vi "Vision_Test.vi"() -> ()   [LabVIEW 2011]
uses:
  <vilib>/Rock Robotics/WPI/Camera/WPI_CameraImageSize.ctl
  <vilib>/Platform/TimedLoop/XDataNode/timing_clust.ctl
  <vilib>/Platform/TimedLoop/XDataNode/nitl_modes.ctl
  <vilib>/Platform/TimedLoop/XDataNode/wakeup.ctl
  <vilib>/Platform/TimedLoop/XDataNode/XDataNode.xnode
  <vilib>/vision/NI_Vision_Development_Module.lvlib
  <vilib>/Platform/TimedLoop/XDataNode/XDNodeRunTimeDep.lvlib
panel:
  out "Wait":bool
  in  "Image Res":T1=enum."320x240"
  out "Offset_Angle_From_Perpendicular":dbl
  out "Shortest_Dist_To_Rect_Center":dbl
  in  "Rect_Width":dbl=24.0
  out "Processed Image":T2(plugin-control)
  out "Raw 2":T2(plugin-control)
  out "Raw 1":T2(plugin-control)
  in  "Threshold Range":cluster{"Lower value":sgl, "Upper value":sgl}={"Lower value"=240.0, "Upper value"=255.0} {"Upper value" format="%.2f"; "Lower value" format="%.2f"}
  out "Image 2":T2(plugin-control)
  out "Image 1":T2(plugin-control)
  in  "Milsec Wait":u32=3000
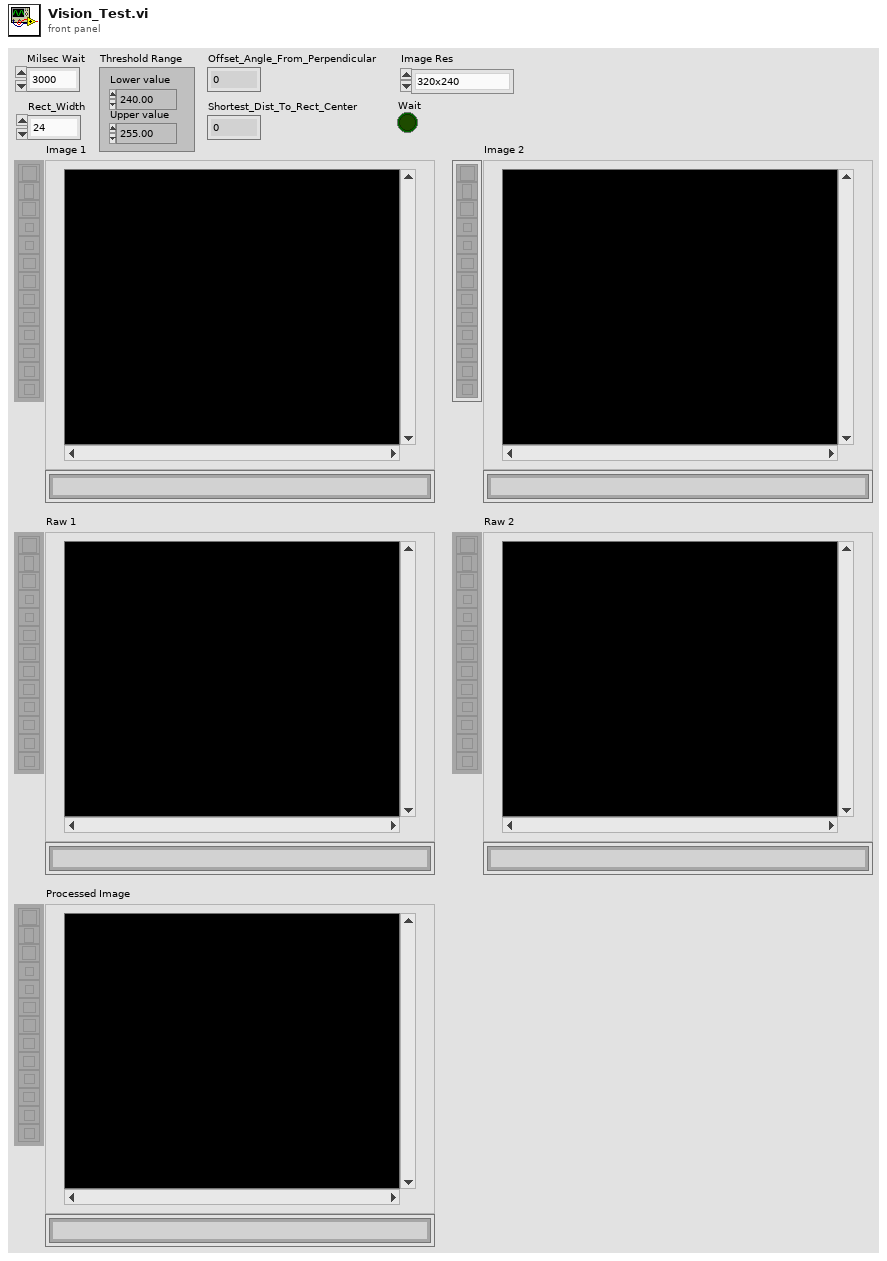
[diagram p1: front panel]
types:
  T1 = typedef "WPI_CameraImageSize.ctl" = enum16{"640x480", "320x240", "160x120"}
  T2 = typedef "IMAQ Image.ctl" = refnum<image>
  T3 = typedef "Image Type" = u32
  T4 = typedef "WPI_CameraDevRef.ctl" = cluster{"Camera Address":string, "CameraStatus":errorcluster, "Acquire Image Notifier":refnum<notifier>}
  T5 = typedef "XDNodeRunTimeDep.lvlib/timing_clust.ctl" = cluster{"Expected End [f-1]":u64, "Actual End [f-1]":u64, "Finished Late? [f-1]":bool, "Expected End [i-1]":u64, "Actual End [i-1]":u64, "Finished Late? [i-1]":bool, "Expected Start [i]":u64, "Actual Start [i]":u64, "Expected Start [f]":u64, "Actual Start [f]":u64, "Source Name":string, "Structure Name":string, "Period":i64, "Deadline":i64, "Offset":i64, "Start":i64, "Priority":i32, "Timeout":i32, "Mode":T6, "Wakeup Reason":T7, "Error":errorcluster, "Source Type":string, "Secondary Source Type":string, "Global End Time":u64, "Global Start Time":u64, "Frame Duration":u64, "Iteration Duration":u64, "Assigned CPU":i32, "I/O Scan Engine Mode":u32}
  T6 = typedef "XDNodeRunTimeDep.lvlib/nitl_modes.ctl" = enum32{"No Change", "Process missed periods, maintain original phase", "Discard missed periods, maintain original phase", "Process missed periods, ignore original phase", "Discard missed periods, ignore original phase"}
  T7 = typedef "XDNodeRunTimeDep.lvlib/wakeup.ctl" = enum32{"Normal", "Aborted", "Asynchronous wakeup", "Timing source error", "Timed loop error", "Timeout"}
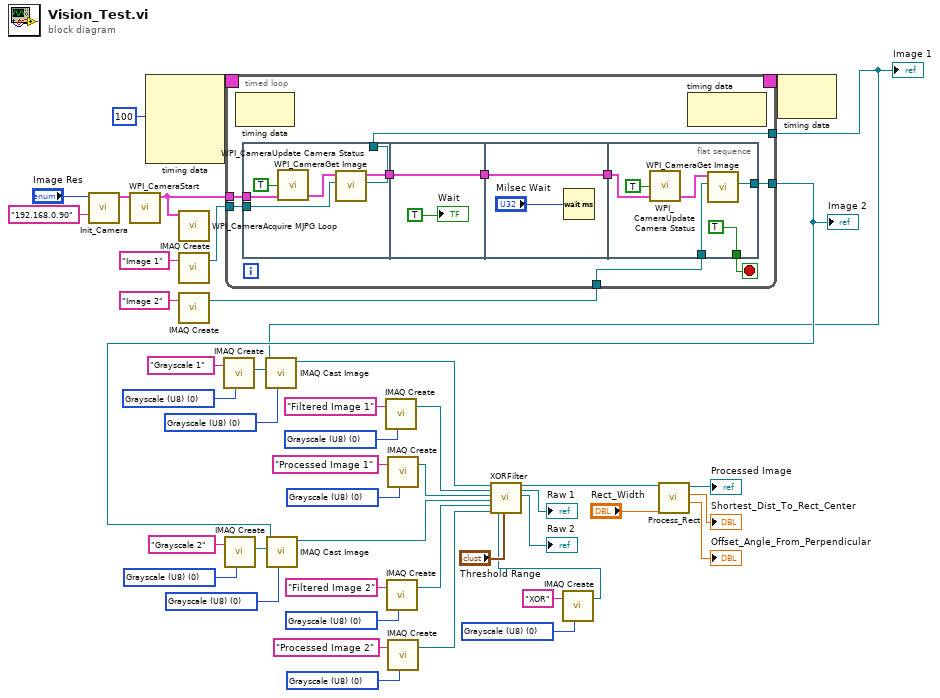
[diagram p0: block diagram]
diagram:
  w17 = T3 0 items=["Grayscale (U8)", "Grayscale (I16)", "Grayscale (SGL)", "Complex (CSG)", "RGB (U32)", "HSL (U32)", "RGB (U64)", "Grayscale (U16)"] ("Image Type")
  w28 = T3 0 items=["Grayscale (U8)", "Grayscale (I16)", "Grayscale (SGL)", "Complex (CSG)", "RGB (U32)", "HSL (U32)", "RGB (U64)", "Grayscale (U16)"] ("Image Type")
  w27 = T3 0 items=["Grayscale (U8)", "Grayscale (I16)", "Grayscale (SGL)", "Complex (CSG)", "RGB (U32)", "HSL (U32)", "RGB (U64)", "Grayscale (U16)"] ("Image Type")
  w29 = T3 0 items=["Grayscale (U8)", "Grayscale (I16)", "Grayscale (SGL)", "Complex (CSG)", "RGB (U32)", "HSL (U32)", "RGB (U64)", "Grayscale (U16)"] ("Image Type")
  w30 = T3 0 items=["Grayscale (U8)", "Grayscale (I16)", "Grayscale (SGL)", "Complex (CSG)", "RGB (U32)", "HSL (U32)", "RGB (U64)", "Grayscale (U16)"] ("Image Type")
  w34 = T3 0 items=["Grayscale (U8)", "Grayscale (I16)", "Grayscale (SGL)", "Complex (CSG)", "RGB (U32)", "HSL (U32)", "RGB (U64)", "Grayscale (U16)"] ("Image Type")
  w35 = T3 0 items=["Grayscale (U8)", "Grayscale (I16)", "Grayscale (SGL)", "Complex (CSG)", "RGB (U32)", "HSL (U32)", "RGB (U64)", "Grayscale (U16)"] ("Image Type")
  w38 = T3 0 items=["Grayscale (U8)", "Grayscale (I16)", "Grayscale (SGL)", "Complex (CSG)", "RGB (U32)", "HSL (U32)", "RGB (U64)", "Grayscale (U16)"] ("Image Type")
  w39 = T3 0 items=["Grayscale (U8)", "Grayscale (I16)", "Grayscale (SGL)", "Complex (CSG)", "RGB (U32)", "HSL (U32)", "RGB (U64)", "Grayscale (U16)"] ("Image Type")
  n1 = call "Init_Camera.vi"("Camera IP"="192.168.0.90", "Image Size"="Image Res") -> ("CameraDevRef Out"=w46:T4)  [unwired: 9 in]
  n2 = call <vilib>:"WPI_CameraStart.vi"("CameraDevRef"=w46) -> ("CameraDevRef Out"=w45:T4)  [unwired: 9 in, 1 out]
  n3 = node-c288(i64 100 ("Period")) -> (w8:T5)  [unwired: 3 in]
  n4 = call <vilib>:"WPI_CameraAcquire MJPG Loop.vi"("CameraDevRef"=w45) -> ()  [unwired: 11 in]
  n5 = call "IMAQ Create"("Image Name"="Image 1") -> ("New Image"=w42:T2)  [unwired: 4 in, 1 out]
  n6 = call "IMAQ Create"("Image Name"="Image 2") -> ("New Image"=w41:T2)  [unwired: 4 in, 1 out]
  n7 = call "IMAQ Create"("Image Name"="Grayscale 1", "Image Type"=w30) -> ("New Image"=w32:T2)  [unwired: 3 in, 1 out]
  n8 = call "IMAQ Create"("Image Name"="Grayscale 2", "Image Type"=w27) -> ("New Image"=w25:T2)  [unwired: 3 in, 1 out]
  n9 = timed-loop {
    tunnel: w45 -> [w54]
    tunnel: w42 -> [w53]
    tunnel: w41 -> [w52]
    tunnel: [w50] -> w24
    timing: w8 -> [_]
    timing-out: [_] -> w7
    tunnel: [w47] -> w4
    stop <- w51 stop-if-true
    n10 = node-c288() -> ()  [unwired: 1 in, 1 out]
    n11 = flat-sequence {
      tunnel: [w61] -> w49
      tunnel: w54 -> [w60]
      tunnel: w53 -> [w59]
      tunnel: [w58] -> _
      tunnel: [w58] -> w47
      tunnel: w49 -> [w65]
      tunnel: [w65] -> w48
      tunnel: [w66] -> w55
      tunnel: w48 -> [w66]
      tunnel: w55 -> [w71]
      tunnel: w52 -> [w70]
      tunnel: [TRUE] -> w51
      tunnel: [w68] -> w50
      frame #0 {
        n12 = call <vilib>:"WPI_CameraUpdate Camera Status.vi"("CameraDevRef In"=w60, "Enable Vision"=TRUE) -> ("CameraDevRef Out"=w63:T4)  [unwired: 3 in]
        n13 = call <vilib>:"WPI_CameraGet Image.vi"("Image"=w59, "CameraDevRef"=w63) -> ("Image Out"=w58:T2, "CameraDevRef Out"=w61:T4)  [unwired: 7 in, 1 out]
      }
      frame #1 {
        "Wait" <- TRUE
      }
      frame #2 {
        n14 = Wait (ms)(milliseconds to wait="Milsec Wait") -> ()  [unwired: 1 out]
      }
      frame #3 {
        n15 = call <vilib>:"WPI_CameraUpdate Camera Status.vi"("CameraDevRef In"=w71, "Enable Vision"=TRUE) -> ("CameraDevRef Out"=w72:T4)  [unwired: 3 in]
        n16 = call <vilib>:"WPI_CameraGet Image.vi"("Image"=w70, "CameraDevRef"=w72) -> ("Image Out"=w68:T2)  [unwired: 7 in, 2 out]
      }
    }
    n17 = node-c288() -> ()  [unwired: 1 in, 1 out]
  }
  "Image 1" <- w4
  "Image 2" <- w24
  n18 = call "IMAQ Cast Image"("Image Type"=w29, "Image Dst"=w32, "Image Src"=w4) -> ("Image Dst Out"=w23:T2)  [unwired: 7 in, 1 out]
  n19 = call "IMAQ Cast Image"("Image Type"=w28, "Image Dst"=w25, "Image Src"=w24) -> ("Image Dst Out"=w20:T2)  [unwired: 7 in, 1 out]
  n20 = call "IMAQ Create"("Image Name"="Filtered Image 1", "Image Type"=w35) -> ("New Image"=w22:T2)  [unwired: 3 in, 1 out]
  n21 = call "IMAQ Create"("Image Name"="Filtered Image 2", "Image Type"=w34) -> ("New Image"=w19:T2)  [unwired: 3 in, 1 out]
  n22 = call "IMAQ Create"("Image Name"="Processed Image 1", "Image Type"=w39) -> ("New Image"=w21:T2)  [unwired: 3 in, 1 out]
  n23 = call "IMAQ Create"("Image Name"="Processed Image 2", "Image Type"=w38) -> ("New Image"=w18:T2)  [unwired: 3 in, 1 out]
  n24 = call "IMAQ Create"("Image Name"="XOR", "Image Type"=w17) -> ("New Image"=w1:T2)  [unwired: 3 in, 1 out]
  n25 = call "XORFilter.vi"("Image Src 1"=w23, "Filtered Image Dst 1"=w22, 2:"Processed Image Dst 2"=w21, "Image Src 2"=w20, "Filtered Image Dst 2"=w19, 5:"Processed Image Dst 2"=w18, "XOR Image Dst"=w1, "Threshold Range"="Threshold Range") -> ("XOR Image Dst Out"=w11:T2, "Image Dst 1 Out"=→"Raw 1":T2, "Image Dst 2 Out"=→"Raw 2":T2)  [unwired: 9 in]
  n26 = call "Process_Rect.vi"("Rect Width"="Rect_Width", "XOR Image"=w11) -> ("Offset Angle From Perpendicular"=→"Offset_Angle_From_Perpendicular":dbl, "Shortest Dist To Rect Center"=→"Shortest_Dist_To_Rect_Center":dbl, "Processed Image Out"=→"Processed Image":T2)  [unwired: 7 in]
  n27 = node-c288(w7) -> ()  [unwired: 1 out]
